vi "Switch Logic.vi"(8 "error in (no error)":T1, 11 "Sim DiscreteIO in":class) -> (0 "error out":T1)   [LabVIEW 2021, in "Sim DiscreteIO.lvclass"]
uses:
  Sim DiscreteIO.lvclass
  C:/Program Files (x86)/National Instruments/LabVIEW 2021/user.lib/S2 Labs/Module Framework/Modules/Base/Module.lvclass
  Sim DiscreteIO.lvclass/Sim DiscreteIO.ctl
  <userlib>/S2 Labs/CVT Toolkit/CVT.lvclass/CVT.ctl
  Accessors/Read Initialized.vi
  8d7a6ccf-5cfe-42ce-bcdb-e88fd19db445.vi
  Accessors/Read occurrence.vi
  8d7a6ccf-5cfe-42ce-bcdb-e88fd19db445.vi/1553f4ce-967c-4f57-a913-5f155bf4374d.vi
  <userlib>/S2 Labs/CVT Toolkit/Read CVT DVR.vi
  <userlib>/S2 Labs/Module Framework/Modules/Base/Get Module CVT Ref.vi
  <vilib>/Utility/error.llb/Error Cluster From Error Code.vi
  <vilib>/rvi/errors/niLvFpgaAdjustHostInterfaceError.vi
  <vilib>/rvi/interface/nirviReadWriteControl/nirviReadWriteControl.xnode
  <userlib>/S2 Labs/Module Framework/Modules/Base/Module.lvclass
  NiFpgaLv.dll
  <vilib>/rvi/interface/Simulation/niFpgaSimulationCallBeginRW.vi
panel:
  out "Stopped?":boolean
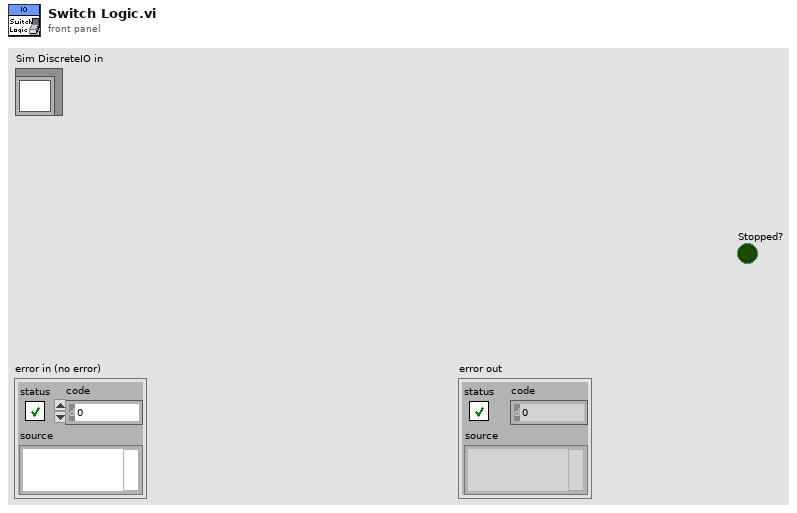
[diagram p1: front panel]
types:
  T1 = cluster{"source":string, "code":numeric, "status":boolean}
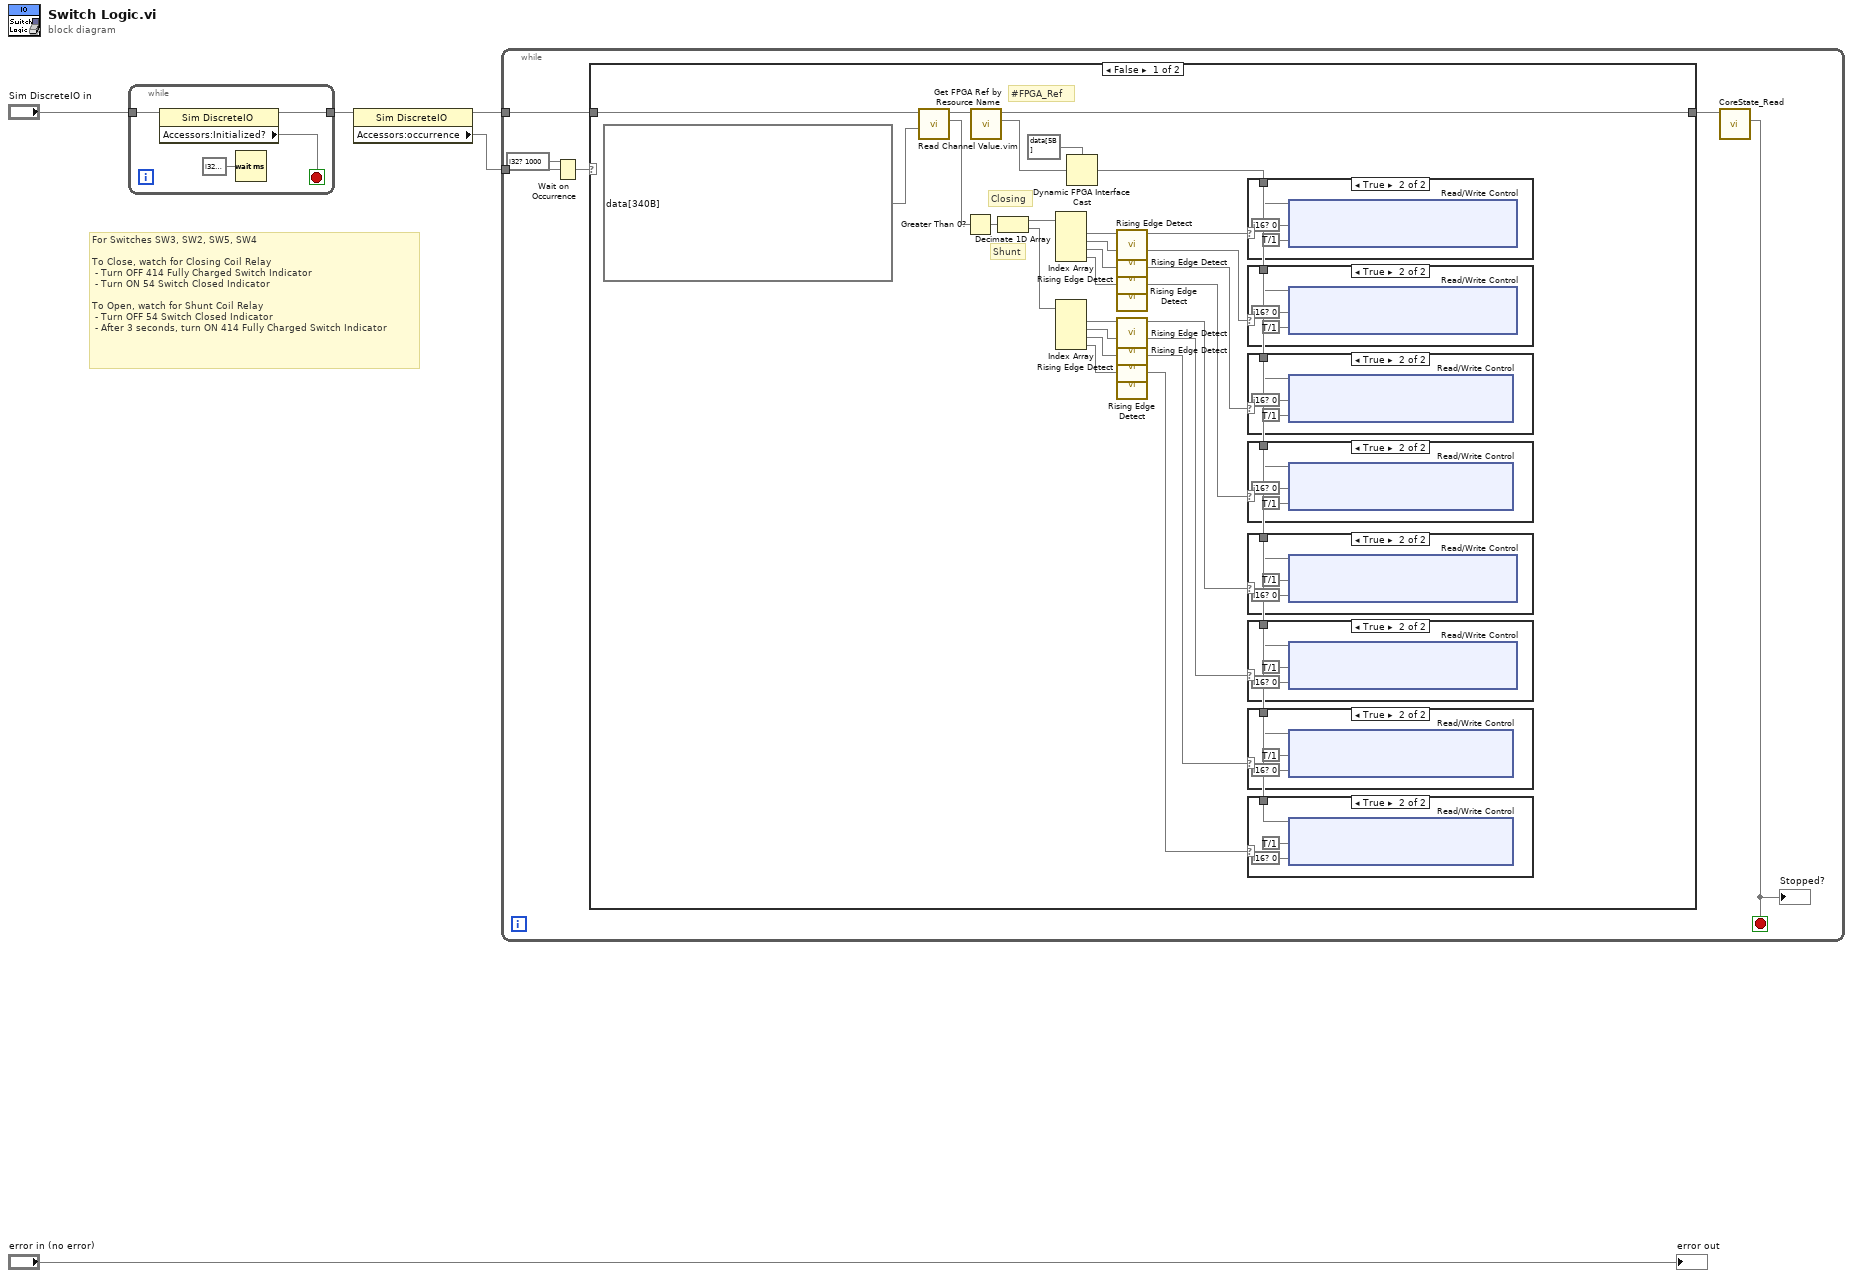
[diagram p0: block diagram]
diagram:
  # "For Switches SW3, SW2, SW5, SW4 \n\nTo Close, watch for Closing Coil Relay\n - Turn OFF 414 Fully Charged Switch Indicator\n - Turn ON 54 Switch Closed Indicator\n\nTo Open, watch for Shunt Coil Relay\n - Turn OFF 54 Switch Closed Indicator\n - After 3 seconds, turn ON 414 Fully Charged Switch Indicator"
  n1 = while {
    tunnel: [w9] -> w3
    tunnel: "Sim DiscreteIO in" -> [w8]
    stop <- w7 stop-if-true
    n2 = property class="Sim DiscreteIO"(reference=w8) -> (reference out=w9, "Accessors:Initialized?"=w7)  [unwired: 1 in, 1 out]
    n3 = Wait (ms)(milliseconds to wait=i32? 100) -> ()  [unwired: 1 out]
  }
  n4 = property class="Sim DiscreteIO"(reference=w3) -> (reference out=w2, "Accessors:occurrence"=w1)  [unwired: 1 in, 1 out]
  n5 = while {
    tunnel: w2 -> [w13]
    tunnel: w1 -> [w12]
    stop <- w15 stop-if-true
    n6 = Wait on Occurrence(2:w12, 3:i32? 1000 ("ms timeout (-1)")) -> (0:w10)  [unwired: 1 in]
    n7 = case shown="False" w10 {
      tunnel: [w25 w67] -> w14
      tunnel: w13 -> [w42 w67]
      frame 0 {
        # "#FPGA_Ref"
        # "Shunt"
        # "Closing"
        n8 = call "Read Channel Value.vim"(9:data[340B] ("Channel Label(s)"), 11:w42) -> (2:w40, 3:w26)  [unwired: 3 in, 5 out]
        n9 = Greater Than 0?(x=w40) -> (x > 0?=w39)
        n10 = call <userlib>:"Get FPGA Ref by Resource Name.vi"(11:w26) -> (2:w28, 3:w25)  [unwired: 7 in, 2 out]
        n11 = Decimate 1D Array(w39) -> (w38, w29)
        n12 = Index Array(array=w38) -> (element #1=w37, element #2=w36, element #3=w35, element #4=w34)  [unwired: 4 in]
        n13 = Index Array(array=w29) -> (element #1=w30, element #2=w31, element #3=w32, element #4=w33)  [unwired: 4 in]
        n14 = Dynamic FPGA Interface Cast(Session In=data[5B] ("Type"), Type=w28) -> (Session Out=w16)
        n15 = call "Rising Edge Detect.vi"(11:w37) -> (3:w24)  [unwired: 10 in]
        n16 = call "Rising Edge Detect.vi"(11:w36) -> (3:w23)  [unwired: 10 in]
        n17 = call "Rising Edge Detect.vi"(11:w35) -> (3:w22)  [unwired: 10 in]
        n18 = call "Rising Edge Detect.vi"(11:w34) -> (3:w21)  [unwired: 10 in]
        n19 = call "Rising Edge Detect.vi"(11:w30) -> (3:w20)  [unwired: 10 in]
        n20 = call "Rising Edge Detect.vi"(11:w31) -> (3:w19)  [unwired: 10 in]
        n21 = call "Rising Edge Detect.vi"(11:w32) -> (3:w18)  [unwired: 10 in]
        n22 = call "Rising Edge Detect.vi"(11:w33) -> (3:w17)  [unwired: 10 in]
        n23 = case shown="True" w24 {
          tunnel: w16 -> [_ w66]
          frame 0 {
          }
          frame 1 {
            n24 = xnode "Read/Write Control"(w66, i16? 0 ("SIM_S1-DI1_AFE1 Disc-Switch SW3 (414)"), T/1 ("SIM_S1-DI0_AFE1 Disc-Switch SW3 (54)")) -> ()  [unwired: 1 in, 2 out]
          }
        }
        n25 = case shown="True" w23 {
          tunnel: w16 -> [_ w63]
          frame 0 {
          }
          frame 1 {
            n26 = xnode "Read/Write Control"(w63, i16? 0 ("SIM_S1-DI1_AFE1 Disc-Switch SW3 (414)"), T/1 ("SIM_S1-DI0_AFE1 Disc-Switch SW3 (54)")) -> ()  [unwired: 1 in, 2 out]
          }
        }
        n27 = case shown="True" w22 {
          tunnel: w16 -> [_ w60]
          frame 0 {
          }
          frame 1 {
            n28 = xnode "Read/Write Control"(w60, i16? 0 ("SIM_S1-DI1_AFE1 Disc-Switch SW3 (414)"), T/1 ("SIM_S1-DI0_AFE1 Disc-Switch SW3 (54)")) -> ()  [unwired: 1 in, 2 out]
          }
        }
        n29 = case shown="True" w21 {
          tunnel: w16 -> [_ w57]
          frame 0 {
          }
          frame 1 {
            n30 = xnode "Read/Write Control"(w57, i16? 0 ("SIM_S1-DI1_AFE1 Disc-Switch SW3 (414)"), T/1 ("SIM_S1-DI0_AFE1 Disc-Switch SW3 (54)")) -> ()  [unwired: 1 in, 2 out]
          }
        }
        n31 = case shown="True" w20 {
          tunnel: w16 -> [_ w54]
          frame 0 {
          }
          frame 1 {
            n32 = xnode "Read/Write Control"(w54, T/1 ("SIM_S1-DI1_AFE1 Disc-Switch SW3 (414)"), i16? 0 ("SIM_S1-DI0_AFE1 Disc-Switch SW3 (54)")) -> ()  [unwired: 1 in, 2 out]
          }
        }
        n33 = case shown="True" w19 {
          tunnel: w16 -> [_ w51]
          frame 0 {
          }
          frame 1 {
            n34 = xnode "Read/Write Control"(w51, T/1 ("SIM_S1-DI1_AFE1 Disc-Switch SW3 (414)"), i16? 0 ("SIM_S1-DI0_AFE1 Disc-Switch SW3 (54)")) -> ()  [unwired: 1 in, 2 out]
          }
        }
        n35 = case shown="True" w18 {
          tunnel: w16 -> [_ w48]
          frame 0 {
          }
          frame 1 {
            n36 = xnode "Read/Write Control"(w48, T/1 ("SIM_S1-DI1_AFE1 Disc-Switch SW3 (414)"), i16? 0 ("SIM_S1-DI0_AFE1 Disc-Switch SW3 (54)")) -> ()  [unwired: 1 in, 2 out]
          }
        }
        n37 = case shown="True" w17 {
          tunnel: w16 -> [_ w45]
          frame 0 {
          }
          frame 1 {
            n38 = xnode "Read/Write Control"(w45, T/1 ("SIM_S1-DI1_AFE1 Disc-Switch SW3 (414)"), i16? 0 ("SIM_S1-DI0_AFE1 Disc-Switch SW3 (54)")) -> ()  [unwired: 1 in, 2 out]
          }
        }
      }
      frame 1 {
      }
    }
    n39 = call-dynamic "CoreState_Read.vi"(11:w14) -> (2:w15)  [unwired: 8 in, 2 out]
    "Stopped?" <- w15
  }
  "error out" <- "error in (no error)"
